vi "GetKnobReference.vi"(8 "error in":errorcluster, 11 "Knob in":refnum<class "Knob.lvclass">) -> (0 "error out":errorcluster, 1 "knob reference":refnum<vi>, 3 "Knob out":refnum<class "Knob.lvclass">)   [LabVIEW 2014, in "Knob.lvclass"]
uses:
  Knob.lvclass
  Generic/Generic.lvclass
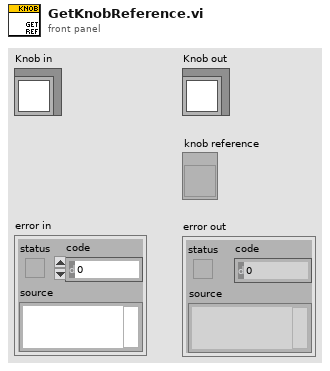
[diagram p1: front panel]
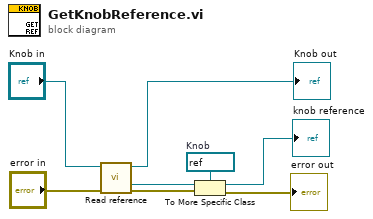
[diagram p0: block diagram]
diagram:
  w2 = refnum<vi> refnum  # Knob
  n1 = call "Read reference.vi"("error in"="error in", "GObject in"="Knob in") -> ("error out"=w6:errorcluster, "reference"=w5:refnum<vi>, "GObject out"=→"Knob out":refnum<class "Knob.lvclass">)  [unwired: 5 in]
  n2 = To More Specific Class(target class=w2, reference=w5, error in=w6) -> (specific class reference=→"knob reference":refnum<vi>, error out=→"error out":errorcluster)
